vi "create color table.vi"() -> ()   [LabVIEW 2009]
panel:
  out "output array":u32[](array[numeric])
  out "Array":u32[][][](array[colorbox])
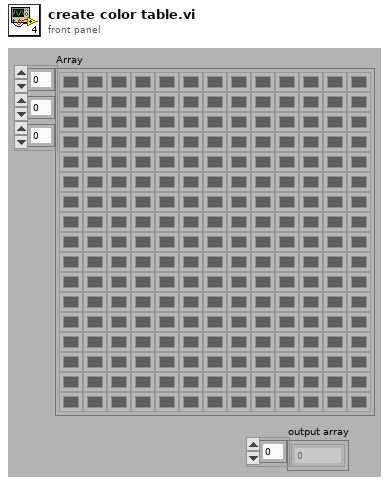
[diagram p1: front panel]
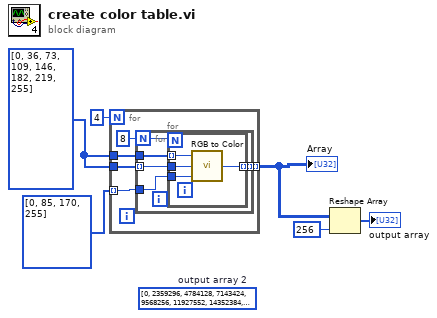
[diagram p0: block diagram]
diagram:
  (unwired) u32[] [0, 2359296, 4784128, 7143424, 9568256, 11927552, 14352384, 16711680, 9216, 2368512, 4793344, 7152640, 9577472, 11936768, 14361600, 16720896, 18688, 2377984, 4802816, 7162112, 9586944, 11946240, 14371072, 16730368, 27904, 2387200, 4812032, 7171328, 9596160, 11955456, 14380288, 16739584, 37376, 2396672, 4821504, 7180800, 9605632, 11964928, 14389760, 16749056, 46592, 2405888, 4830720, 7190016, 9614848, 11974144, 14398976, 16758272, 56064, 2415360, 4840192, 7199488, 9624320, 11983616, 14408448, 16767744, 65280, 2424576, 4849408, 7208704, 9633536, 11992832, 14417664, 16776960, 85, 2359381, 4784213, 7143509, 9568341, 11927637, 14352469, 16711765, 9301, 2368597, 4793429, 7152725, 9577557, 11936853, 14361685, 16720981, 18773, 2378069, 4802901, 7162197, 9587029, 11946325, 14371157, 16730453, 27989, 2387285, 4812117, 7171413, 9596245, 11955541, 14380373, 16739669, 37461, 2396757, 4821589, 7180885, 9605717, 11965013, 14389845, 16749141, 46677, 2405973, 4830805, 7190101, 9614933, 11974229, 14399061, 16758357, 56149, 2415445, 4840277, 7199573, 9624405, 11983701, 14408533, 16767829, 65365, 2424661, 4849493, 7208789, 9633621, 11992917, 14417749, 16777045, 170, 2359466, 4784298, 7143594, 9568426, 11927722, 14352554, 16711850, 9386, 2368682, 4793514, 7152810, 9577642, 11936938, 14361770, 16721066, 18858, 2378154, 4802986, 7162282, 9587114, 11946410, 14371242, 16730538, 28074, 2387370, 4812202, 7171498, 9596330, 11955626, 14380458, 16739754, 37546, 2396842, 4821674, 7180970, 9605802, 11965098, 14389930, 16749226, 46762, 2406058, 4830890, 7190186, 9615018, 11974314, 14399146, 16758442, 56234, 2415530, 4840362, 7199658, 9624490, 11983786, 14408618, 16767914, 65450, 2424746, 4849578, 7208874, 9633706, 11993002, 14417834, 16777130, 255, 2359551, 4784383, 7143679, 9568511, 11927807, 14352639, 16711935, 9471, 2368767, 4793599, 7152895, 9577727, 11937023, 14361855, 16721151, 18943, 2378239, 4803071, 7162367, 9587199, 11946495, 14371327, 16730623, 28159, 2387455, 4812287, 7171583, 9596415, 11955711, 14380543, 16739839, 37631, 2396927, 4821759, 7181055, 9605887, 11965183, 14390015, 16749311, 46847, 2406143, 4830975, 7190271, 9615103, 11974399, 14399231, 16758527, 56319, 2415615, 4840447, 7199743, 9624575, 11983871, 14408703, 16767999, 65535, 2424831, 4849663, 7208959, 9633791, 11993087, 14417919, 16777215]  # output array 2
  w5 = u8[] [0, 36, 73, 109, 146, 182, 219, 255] ("Array")
  n1 = for {
    N: 4 -> [_]
    tunnel: u8[] [0, 85, 170, 255] ("Array") -> [w11] mode=indexing
    tunnel: w5 -> [w10]
    tunnel: w5 -> [w9]
    tunnel: [w8] -> w4 mode=indexing
    n2 = for {
      N: 8 -> [w12]
      tunnel: w11 -> [w16]
      tunnel: w10 -> [w15] mode=indexing
      tunnel: w9 -> [w14]
      tunnel: [w13] -> w8 mode=indexing
      n3 = for {
        N: w12 -> [_]
        tunnel: w16 -> [w20]
        tunnel: w15 -> [w19]
        tunnel: w14 -> [w18] mode=indexing
        tunnel: [w17] -> w13 mode=indexing
        n4 = call <vilib>:"RGB to Color.vi"("B"=w20, "G"=w19, "R"=w18) -> ("Color"=w17:u32)
      }
    }
  }
  "Array" <- w4
  n5 = Reshape Array(w4, 256 ("dimension size")) -> (→"output array":u32[])
